vi "Read Rank.vi"(8 "error in":errorcluster, 11 "SG 26GHz Path Group in":refnum<class "SG 26GHz Path Group.lvclass">) -> (0 "error out":errorcluster, 2 "Rank":dbl, 3 "SG 26GHz Path Group out":refnum<class "SG 26GHz Path Group.lvclass">)   [LabVIEW 2023, in "RFFixtureCharact.PXI.lvlib" / "SG 26GHz Path Group.lvclass"]
uses:
  SG 26GHz Path Group.lvclass
  SG 26GHz Path Group.lvclass/SG 26GHz Path Group.ctl
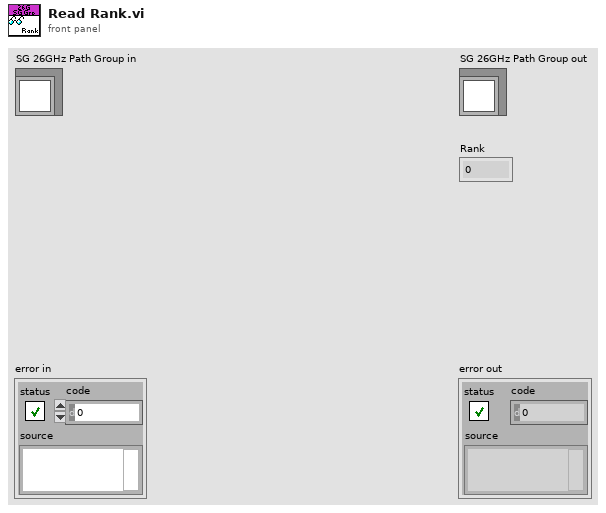
[diagram p1: front panel]
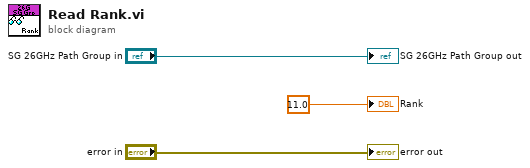
[diagram p0: block diagram]
diagram:
  "error out" <- "error in"
  "SG 26GHz Path Group out" <- "SG 26GHz Path Group in"
  "Rank" <- 11.0 ("Rank")
